vi "Stop recording.vi"() -> ()   [LabVIEW 2014]
panel:
  in  "standard input":string
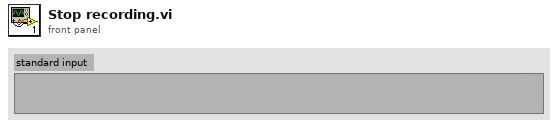
[diagram p1: front panel]
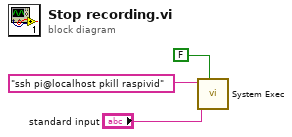
[diagram p0: block diagram]
diagram:
  n1 = call <vilib>:"System Exec.vi"("wait until completion? (T)"=FALSE, "standard input"="standard input", "command line"="ssh pi@localhost pkill raspivid") -> ()  [unwired: 5 in, 4 out]
